vi "KundtsTubeJ&J.vi"() -> ()   [LabVIEW 2015]
panel:
  out "Array":dbl[](array[numeric])
  out "Waveform Graph 2":dynamicdata(graph)
  out "Numeric":i32
  out "element":dbl
  out "Frequency":dbl
  in  "stop":bool
  in  "Tab Control":enum32{"Sweep", "Signal"}(tab)
  in  "milliseconds to wait":u32
  in  "Frequency":dbl
  out "(Vrms)":dbl format="%0.2f"
  in  "Sampling Rate":dbl
  in  "#of Samples":dbl
  out "XY Graph":cluster{dbl[], dbl[]}(graph)
  in  "Cluster":T1
  in  "Amplitude":dbl
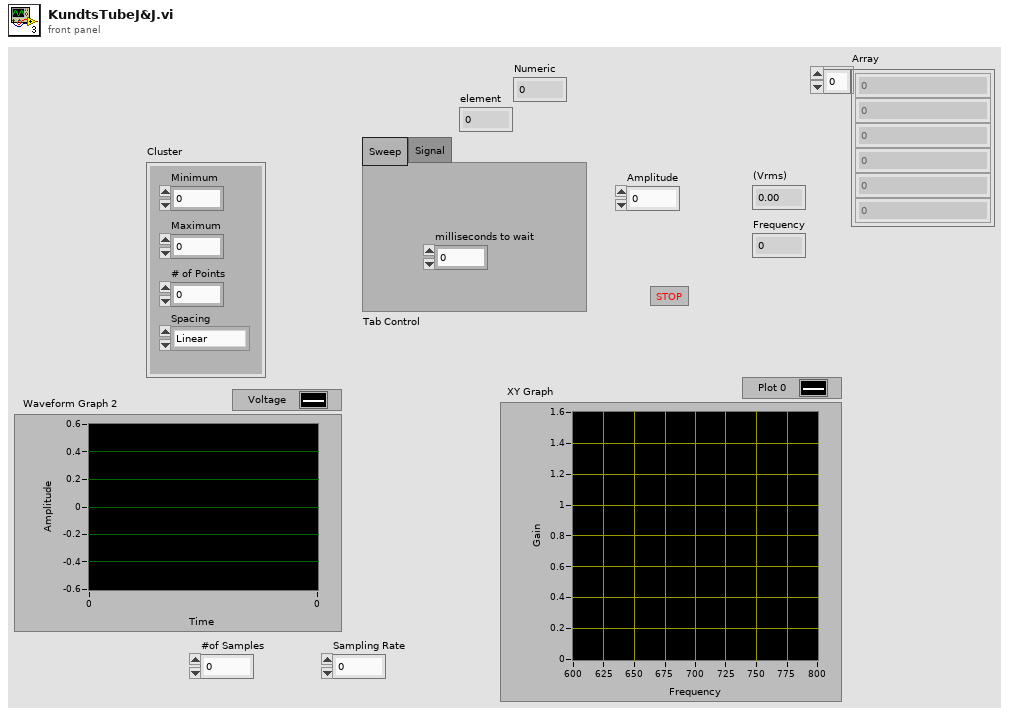
[diagram p1: front panel]
types:
  T1 = cluster{"Minimum":dbl, "Maximum":dbl, "# of Points":dbl, "Spacing":enum16{"Linear", "Logarithmic"}}
  T2 = enum16{"open", "replace", "create", "open or create", "replace or create", "replace or create with confirmation"}
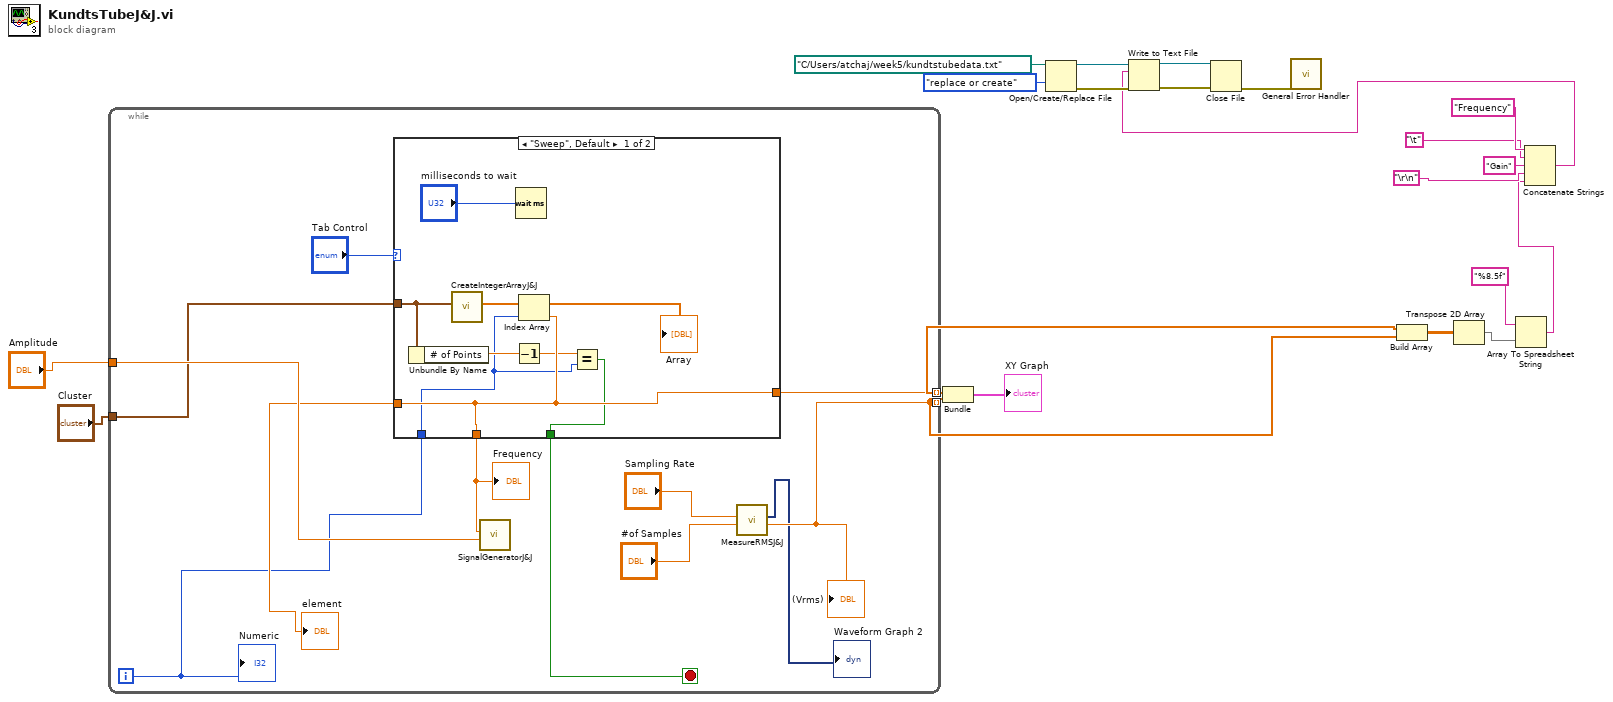
[diagram p0: block diagram]
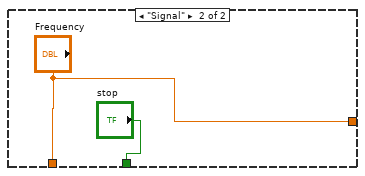
[diagram p2: hidden frame]
diagram:
  n1 = while {
    tunnel: "Amplitude" -> [w32]
    tunnel: [w27] -> w2 mode=indexing
    tunnel: "Cluster" -> [w25]
    tunnel: [w23] -> w1 mode=indexing
    i -> [w24]
    stop <- w30 stop-if-true
    n2 = case shown="\"Sweep\", Default" "Tab Control" {
      tunnel: [w39 "Frequency"] -> w31
      tunnel: [w34 "stop"] -> w30
      tunnel: [w39 _] -> w26
      tunnel: [w39 "Frequency"] -> w27
      tunnel: w25 -> [w38 _]
      tunnel: w24 -> [w35 _]
      frame "Sweep", Default {
        n3 = Unbundle By Name(w38) -> ("# of Points"=w37:dbl)
        n4 = call "CreateIntegerArrayJ&J.vi"("Cluster"=w38) -> ("Array"=w40:dbl[])  [unwired: 10 in]
        "Array" <- w40
        n5 = Decrement(x=w37) -> (x-1=w36:dbl)
        n6 = Wait (ms)(milliseconds to wait="milliseconds to wait") -> ()  [unwired: 1 out]
        n7 = Index Array(array=w40, index=w35) -> (element=w39:dbl)
        n8 = Equal?(x=w36, y=w35) -> (x = y?=w34:bool)
      }
      frame "Signal" {
      }
    }
    "Frequency" <- w31
    "element" <- w26
    n9 = call "SignalGeneratorJ&J.vi"("Amplitude"=w32, "Frequency"=w31) -> ()  [unwired: 10 in]
    n10 = call "MeasureRMSJ&J.vi"("#of Samples"="#of Samples", "Sampling Rate"="Sampling Rate") -> ("(Vrms)"=w23:dbl, "Waveform Graph"=→"Waveform Graph 2":dynamicdata)  [unwired: 8 in]
    "(Vrms)" <- w23
    "Numeric" <- w24
  }
  n11 = Bundle(w2, w1) -> (→"XY Graph":cluster{dbl[], dbl[]})  [unwired: 1 in]
  n12 = Open/Create/Replace File(file path (use dialog)=path "C:/Users/atchaj/week5/kundtstubedata.txt", operation (0:open)=T2."replace or create") -> (refnum out=w15:refnum<file>, error out=w16:errorcluster)  [unwired: 4 in, 1 out]
  n13 = Build Array(w2, w1) -> (w10:dbl[][])
  n14 = Transpose 2D Array(2D array=w10) -> (transposed array=w11:dbl[][])
  n15 = Array To Spreadsheet String(array=w11, 3:"%8.5f" ("format string")) -> (spreadsheet string=w5:string)  [unwired: 1 in]
  n16 = Concatenate Strings("Frequency" ("string"), "\t", "Gain" ("string"), "\r\n", w5) -> (w4:string)
  n17 = Write to Text File(file (use dialog)=w15, text=w4, error in=w16) -> (refnum out=w14:refnum<file>, error out=w17:errorcluster)  [unwired: 1 in, 1 out]
  n18 = Close File(refnum=w14, error in=w17) -> (error out=w18:errorcluster)  [unwired: 1 out]
  n19 = call <vilib>:"General Error Handler.vi"("error in (no error)"=w18) -> ()  [unwired: 10 in, 5 out]
